vi "CHD_ODOM_DASH_WRITE.vi"   [LabVIEW 2019]
uses:
  CHD_ODOM_GLOBALS.vi
  <vilib>/Rock Robotics/Network Tables/NT Write Number.vi
types:
  T1 = typedef "Trajectory_Library.lvlib/POSE2D.ctl" = cluster{"TRANSLATION":T2, "ROTATION":T3}
  T2 = typedef "Trajectory_Library.lvlib/TRANSLATION2D.ctl" = cluster{"X":dbl, "Y":dbl}
  T3 = typedef "Trajectory_Library.lvlib/ROTATION2D.ctl" = cluster{"VALUE":dbl, "COS":dbl, "SIN":dbl}
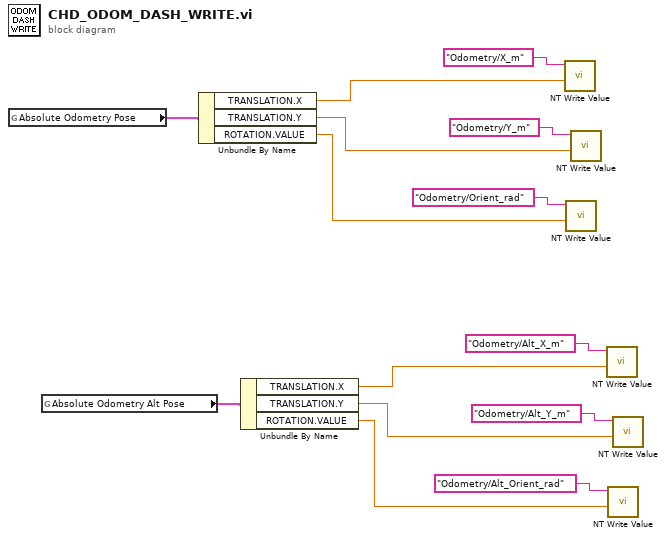
[diagram p0: block diagram]
diagram:
  n1 = global read "CHD_ODOM_GLOBALS.vi" "Absolute Odometry Pose"() -> (w11:T1)
  n2 = global read "CHD_ODOM_GLOBALS.vi" "Absolute Odometry Alt Pose"() -> (w4:T1)
  n3 = Unbundle By Name(w11) -> ("TRANSLATION.X"=w10:dbl, "TRANSLATION.Y"=w9:dbl, "ROTATION.VALUE"=w8:dbl)
  n4 = Unbundle By Name(w4) -> ("TRANSLATION.X"=w3:dbl, "TRANSLATION.Y"=w2:dbl, "ROTATION.VALUE"=w1:dbl)
  n5 = call-poly <vilib>:"NT Write Value.vi"("value"=w10, "name"="Odometry/X_m" ("Name")) -> ()  [unwired: 9 in, 1 out]
  n6 = call-poly <vilib>:"NT Write Value.vi"("value"=w8, "name"="Odometry/Orient_rad" ("Name")) -> ()  [unwired: 9 in, 1 out]
  n7 = call-poly <vilib>:"NT Write Value.vi"("value"=w9, "name"="Odometry/Y_m" ("Name")) -> ()  [unwired: 9 in, 1 out]
  n8 = call-poly <vilib>:"NT Write Value.vi"("value"=w3, "name"="Odometry/Alt_X_m" ("Name")) -> ()  [unwired: 9 in, 1 out]
  n9 = call-poly <vilib>:"NT Write Value.vi"("value"=w1, "name"="Odometry/Alt_Orient_rad" ("Name")) -> ()  [unwired: 9 in, 1 out]
  n10 = call-poly <vilib>:"NT Write Value.vi"("value"=w2, "name"="Odometry/Alt_Y_m" ("Name")) -> ()  [unwired: 9 in, 1 out]
